vi "LHF.DB.Mongo.Collection.RemoveById.vi"(8 "error in (no error)":errorcluster, 9 "_id":string, 10 "collectionName":string, 11 "LHF.DB.Mongo in":refnum<class "LHF.DB.Mongo.lvclass">) -> (0 "error out":errorcluster, 3 "LHF.DB.Mongo out":refnum<class "LHF.DB.Mongo.lvclass">)   [LabVIEW 2013, in "LHF.DB.Mongo.lvclass"]
uses:
  LHF.DB.Mongo.lvclass
  C:/Users/Ricardo/Desktop/Projetos/LabVIEW-MongoDB/src/Driver/MongoDB.Bson.dll
  LabVIEW-MongoDB/src/Driver/MongoDB.Bson.dll
  C:/Users/Ricardo/Desktop/Projetos/LabVIEW-MongoDB/src/Driver/MongoDB.Driver.dll
  LabVIEW-MongoDB/src/Driver/MongoDB.Driver.dll
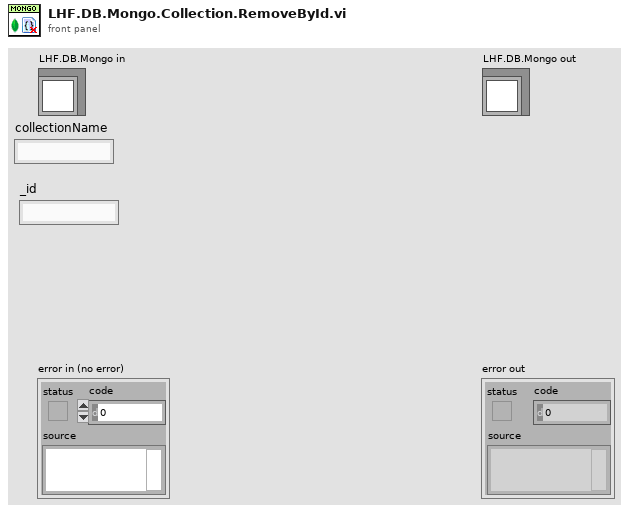
[diagram p1: front panel]
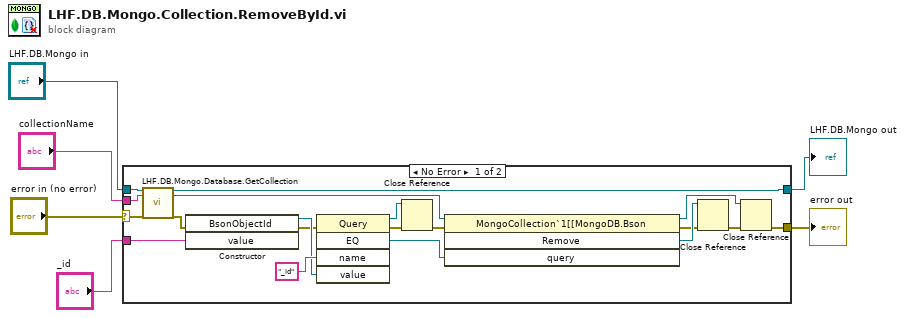
[diagram p0: block diagram]
diagram:
  n1 = case shown="No Error" "error in (no error)" {
    selector: "error in (no error)" -> [w12 w27]
    tunnel: [w20 w26] -> w4
    tunnel: "LHF.DB.Mongo in" -> [w21 w26]
    tunnel: "collectionName" -> [w22 _]
    tunnel: "_id" -> [w19 _]
    tunnel: [w8 w27] -> w1
    frame No Error {
      n2 = call "LHF.DB.Mongo.Database.GetCollection.vi"("LHF.DB.Mongo in"=w21, "collectionName"=w22, "error in (no error)"=w12) -> ("LHF.DB.Mongo in"=w20:refnum<class "LHF.DB.Mongo.lvclass">, "MongoCollection"=w16:refnum<k24>, "error out"=w15:errorcluster)  [unwired: 14 in]
      n3 = constructor class="BsonObjectId"(error in=w15, "value"=w19) -> (reference out=w18:refnum<k24>, error out=w14:errorcluster)  [unwired: 2 in, 2 out]
      n4 = invoke class="Query" method="EQ"(error in=w14, "name"="_id", "value"=w18) -> (reference out=w24:refnum<k24>, error out=w23:errorcluster, "EQ"=w17:refnum<k24>)  [unwired: 2 in, 2 out]
      n5 = Close Reference(reference=w24, error in (no error)=w23) -> (error out=w7:errorcluster)
      n6 = invoke class="MongoCollection`1[[MongoDB.Bson" method="Remove"(reference=w16, error in=w7, "query"=w17) -> (reference out=w11:refnum<k24>, error out=w10:errorcluster, "Remove"=w13:refnum<k24>)  [unwired: 1 in, 1 out]
      n7 = Close Reference(reference=w13, error in (no error)=w10) -> (error out=w9:errorcluster)
      n8 = Close Reference(reference=w11, error in (no error)=w9) -> (error out=w8:errorcluster)
    }
    frame Error {
    }
  }
  "error out" <- w1
  "LHF.DB.Mongo out" <- w4
